vi "Write Size.vi"(8 "error in (no error)":errorcluster, 10 "Size":enum16{"Small", "Middle", "Big"}(ring), 11 "UIStep in":refnum<class "UIStep.lvclass">) -> (0 "error out":errorcluster, 3 "UIStep out":refnum<class "UIStep.lvclass">)   [LabVIEW 2015, in "UIStep.lvclass"]
uses:
  UIStep.lvclass
  UIStep.lvclass/UIStep.ctl
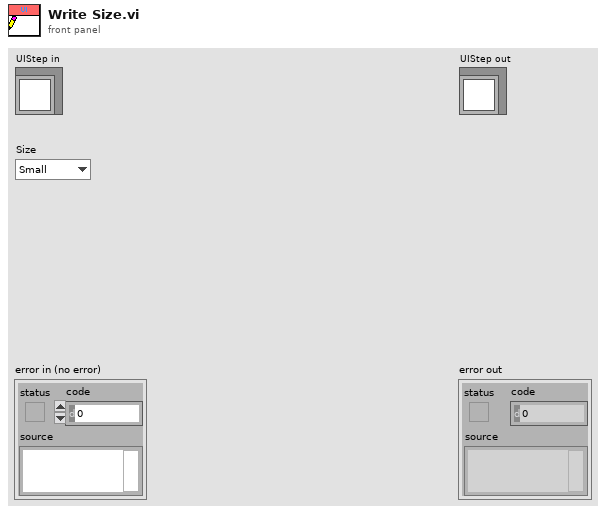
[diagram p1: front panel]
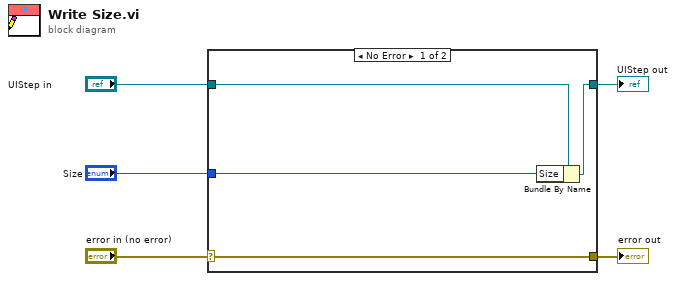
[diagram p0: block diagram]
diagram:
  n1 = case shown="No Error" "error in (no error)" {
    selector: "error in (no error)" -> [w9 w10]
    tunnel: [w9 w10] -> w4
    tunnel: [w7 w11] -> w2
    tunnel: "UIStep in" -> [w8 w11]
    tunnel: "Size" -> [w6 _]
    frame No Error {
      n2 = Bundle By Name(cluster=w8, "Size"=w6) -> (w7:refnum<class "UIStep.lvclass">)
    }
    frame Error {
    }
  }
  "error out" <- w4
  "UIStep out" <- w2
